vi "HeatPropagationStep.vi"(7 "error in (no error)":errorcluster, 8 "liquid":T4, 9 "heater":T3, 10 "tank":T2) -> (0 "error out":errorcluster, 1 "Y Scale":T1, 2 "X Scale":T1, 3 "next_temperature":dbl[][](array[numeric]))   [LabVIEW 2020]
uses:
  Liquid.ctl
  Heater.ctl
  TankResolution.ctl
  <vilib>/Utility/miscctls.llb/LVOffsetAndMultiplierTypeDef.ctl
  <vilib>/gmath/pde.llb/Define 2D Heat PDE IC (Numeric).vi
  <vilib>/gmath/pde.llb/2D Heat PDE Solver (Rect Domain).vi
  <vilib>/gmath/pde.llb/2D Heat PDE Rendering (Rect Domain).vi
  <vilib>/gmath/NI_PDE.lvlib
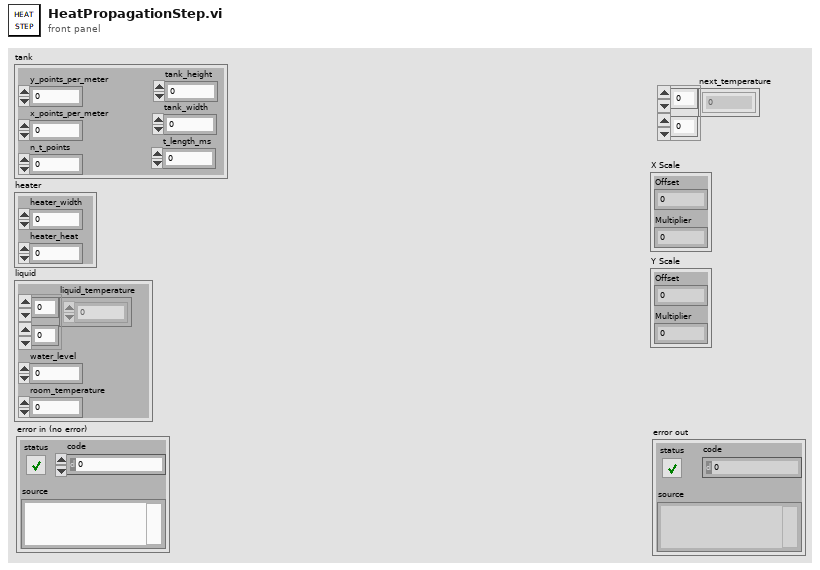
[diagram p1: front panel]
types:
  T1 = typedef "LVOffsetAndMultiplierTypeDef.ctl" = cluster{"Offset":dbl, "Multiplier":dbl}
  T2 = typedef "TankResolution.ctl" = cluster{"y_points_per_meter":i32, "x_points_per_meter":i32, "n_t_points":i32, "tank_height":dbl, "tank_width":dbl, "t_length_ms":u32}
  T3 = typedef "Heater.ctl" = cluster{"heater_width":dbl, "heater_heat":dbl}
  T4 = typedef "Liquid.ctl" = cluster{"liquid_temperature":dbl[][], "water_level":dbl, "room_temperature":dbl}
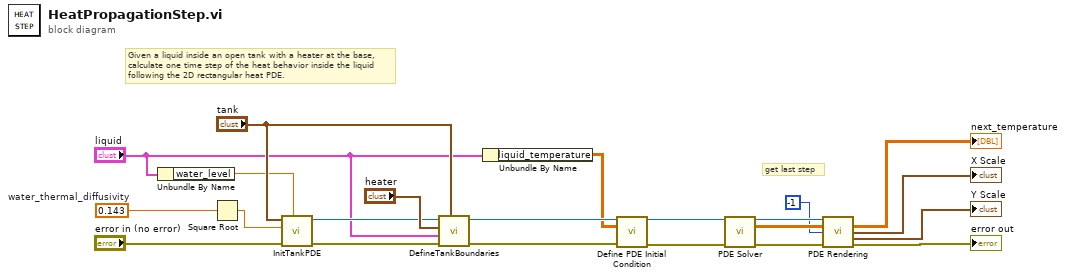
[diagram p0: block diagram]
diagram:
  w4 = 0.143  # water_thermal_diffusivity
  # "Given a liquid inside an open tank with a heater at the base, calculate one time step of the heat behavior inside the liquid following the 2D rectangular heat PDE."
  # "get last step"
  n1 = Unbundle By Name("liquid") -> ("water_level"=w5:dbl)
  n2 = Square Root(x=w4) -> (sqrt(x)=w3:dbl)
  n3 = call "InitTankPDE.vi"("water_level"=w5, "error in (no error)"="error in (no error)", "k"=w3, "tank_resolution"="tank") -> ("error out"=w22:errorcluster, "PDE out"=w17:refnum<class "NI_PDE.lvclass">)  [unwired: 6 in]
  n4 = call "DefineTankBoundaries.vi"("tank_resolution"="tank", "error in (no error)"=w22, "liquid"="liquid", "heater"="heater", "PDE in"=w17) -> ("error out"=w15:errorcluster, "PDE out"=w16:refnum<class "NI_PDE.lvclass">)  [unwired: 5 in]
  n5 = Unbundle By Name("liquid") -> ("liquid_temperature"=w2:dbl[][])
  n6 = call-poly <vilib>:"Define PDE Initial Condition.vi"("PDE in"=w16, "Initial Condition"=w2, "error in (no error)"=w15) -> ("PDE out"=w6:refnum<class "NI_PDE.lvclass">, "error out"=w7:errorcluster)  [unwired: 11 in]
  n7 = call-poly <vilib>:"PDE Solver.vi"("PDE in"=w6, "error in (no error)"=w7) -> ("PDE out"=w9:refnum<class "NI_PDE.lvclass">, "U(t, x, y)"=w14:dbl[][][], "error out"=w10:errorcluster)  [unwired: 11 in]
  n8 = call-poly <vilib>:"PDE Rendering.vi"("PDE in"=w9, "U(t, x, y)"=w14, "index (time step)"=-1, "error in (no error)"=w10) -> ("PDE Plot"=→"next_temperature":dbl[][], "X Scale"=→"X Scale":T1, "Y Scale"=→"Y Scale":T1, "error out"=→"error out":errorcluster)  [unwired: 7 in, 1 out]
